vi "Get File Extension.vi"(8 "error in (no error)":errorcluster, 11 "MusicFile":refnum<class "MusicFile.lvclass">) -> (0 "error out":errorcluster, 2 "File Extention":string, 3 "MusicFile":refnum<class "MusicFile.lvclass">)   [LabVIEW 2015, in "MusicFile.lvclass"]
uses:
  MusicFile.lvclass
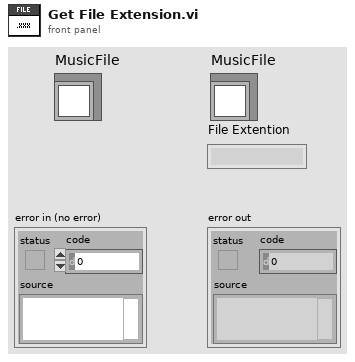
[diagram p1: front panel]
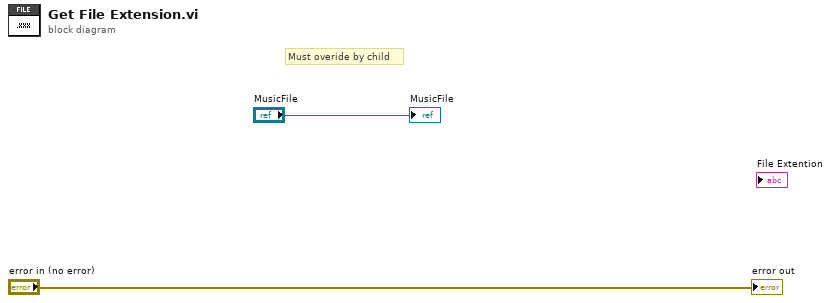
[diagram p0: block diagram]
diagram:
  # "Must overide by child"
  "error out" <- "error in (no error)"
  "MusicFile" <- "MusicFile"
